vi "p1.vi"() -> ()   [LabVIEW 2023, in "d19.lvlib"]
uses:
  d19.lvlib
  AOC/AOC.lvlib
panel:
  in  "Example":string
  in  "Example":bool=TRUE
  out "Answer":i32=978
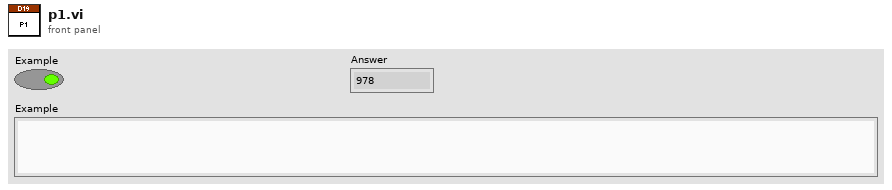
[diagram p1: front panel]
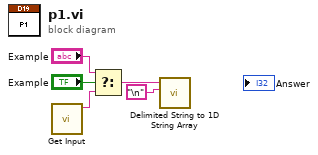
[diagram p0: block diagram]
diagram:
  n1 = call "Get Input.vi"() -> ("Input"=w5:string)  [unwired: 11 in]
  n2 = Select(t="Example", s="Example", f=w5) -> (s? t:f=w4:string)
  n3 = call <vilib>:"Delimited String to 1D String Array.vi"("delimiter"="\n", "delimited string"=w4) -> ()  [unwired: 9 in, 1 out]
